vi "DF_conveyer_belt_control.vi"() -> ()   [LabVIEW 2019]
uses:
  LabVIEW_LJM/FoamWood/Control 3.ctl
  <vilib>/Instr/_visa.llb/VISA Configure Serial Port (Instr).vi
panel:
  in  "stop":bool
  in  "Speed (Hz)":T1=-5.5 step=0.1 format="%#_4g"
  in  "COM port":refnum<visa-resource-name>="COM7"
  out "error out":errorcluster={"status"=FALSE, "code"=1073676294, "source"="VISA Read in DF_conveyer_belt_control.vi"}
  # "Speed of the conveyer belt. The sign define the direction of the rotation."
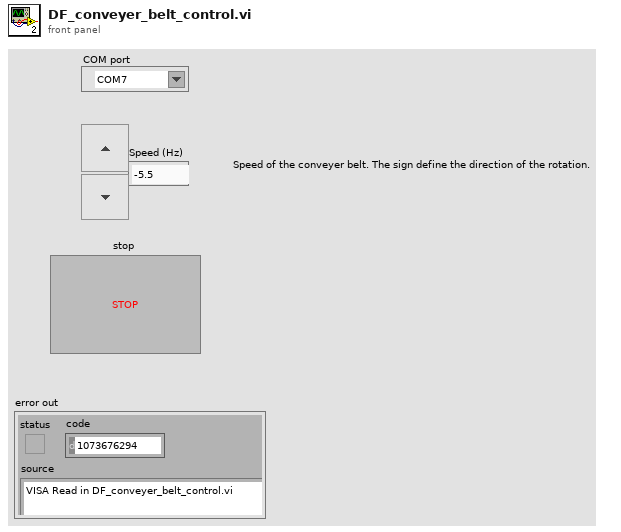
[diagram p1: front panel]
types:
  T1 = typedef "Control 3.ctl" = dbl
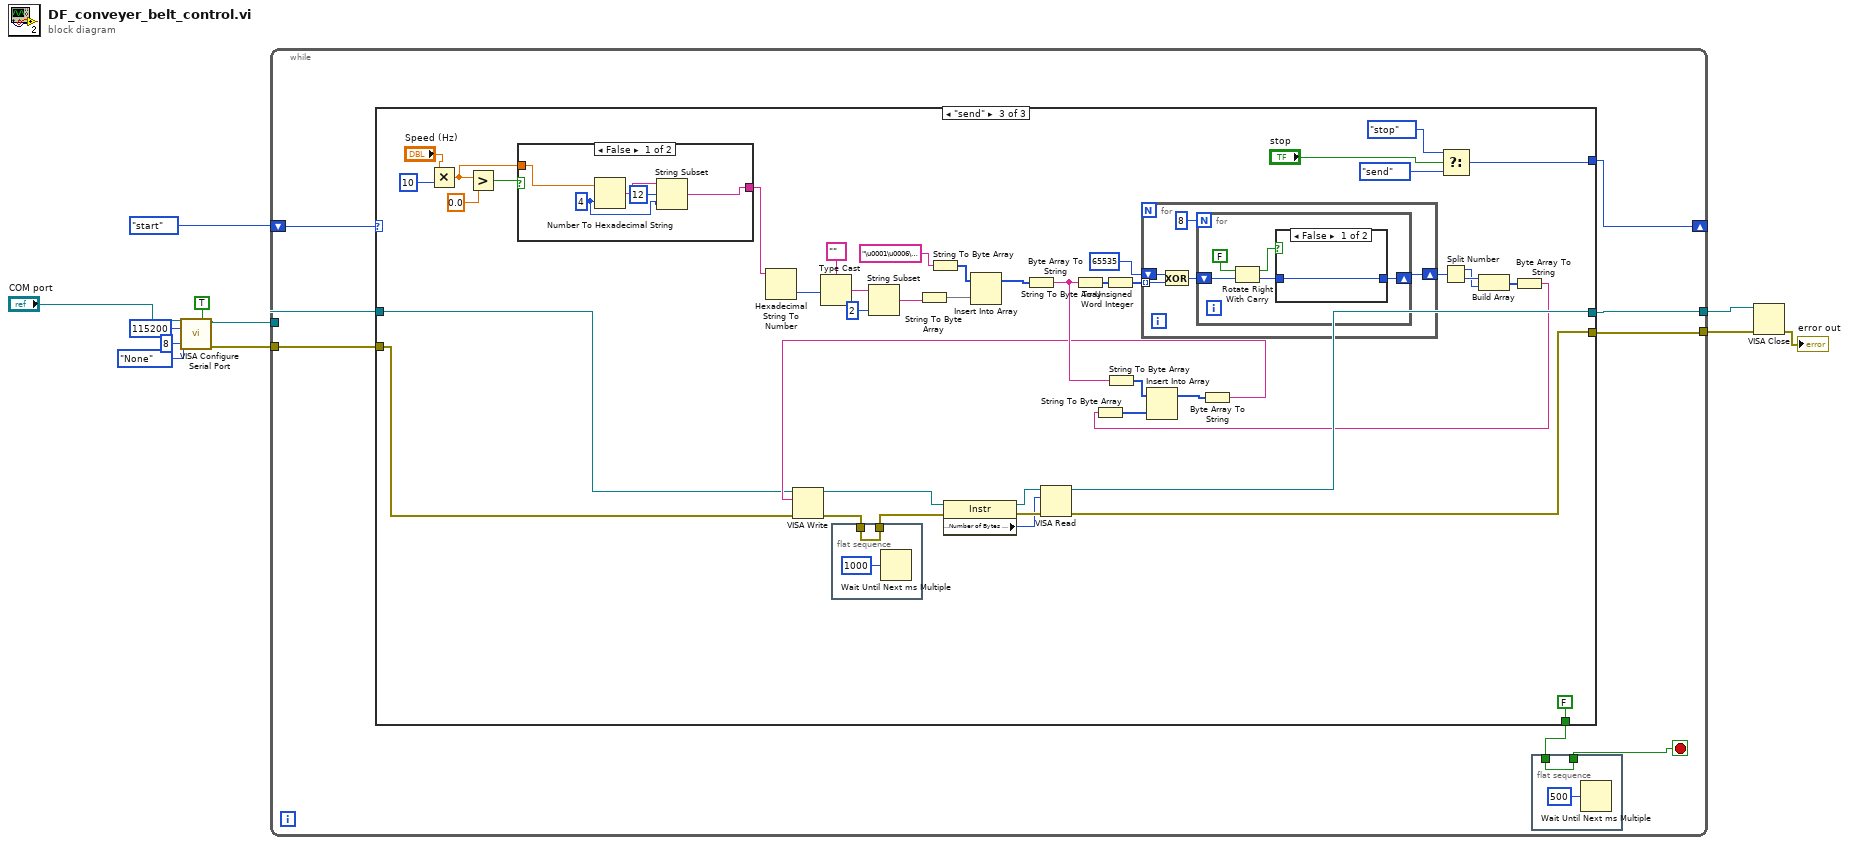
[diagram p0: block diagram]
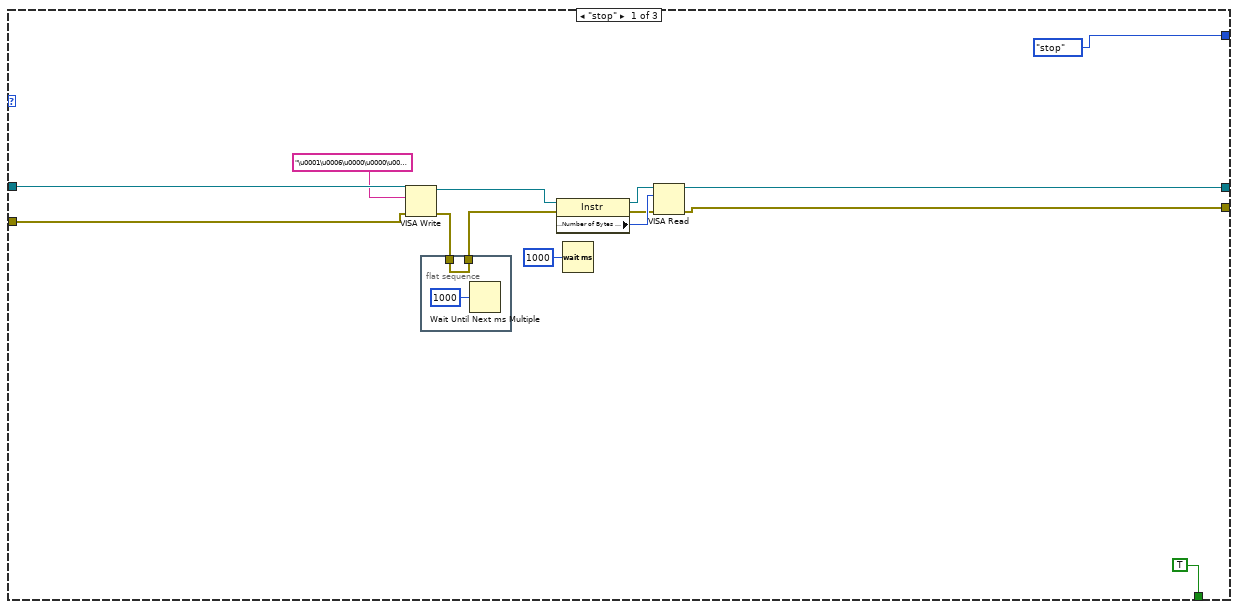
[diagram p2: hidden frame]
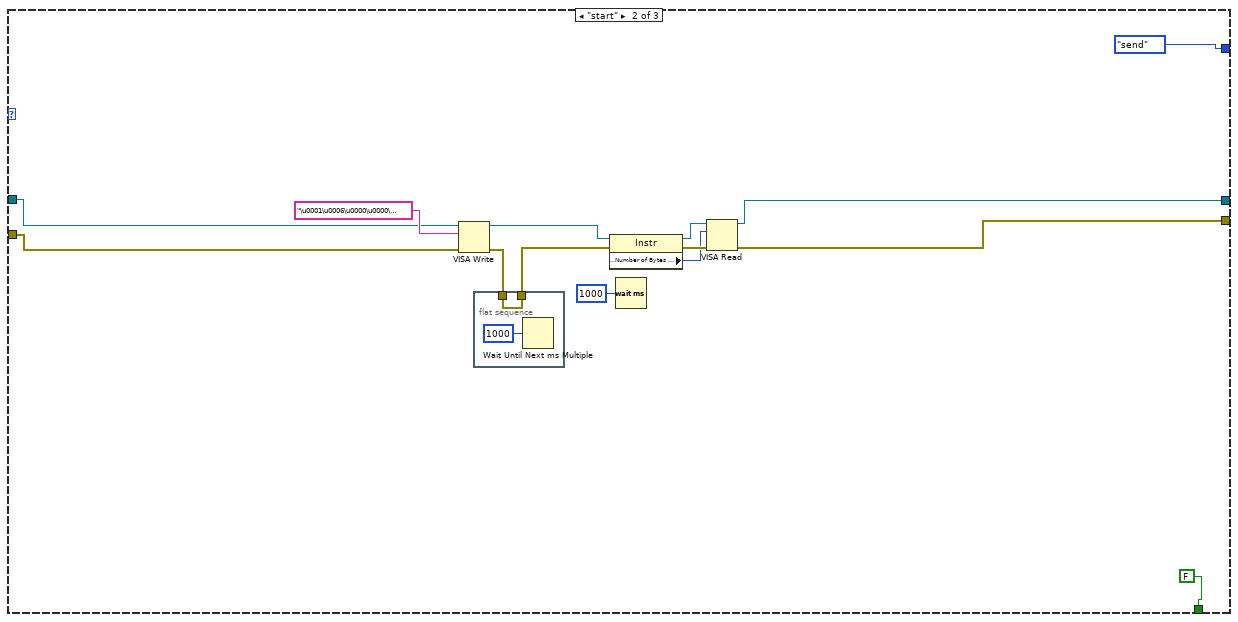
[diagram p3: hidden frame]
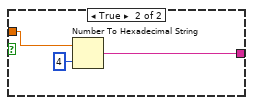
[diagram p4: hidden frame]
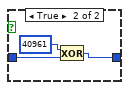
[diagram p5: hidden frame]
diagram:
  n1 = call-poly "VISA Configure Serial Port"("VISA resource name"="COM port", "Enable Termination\nChar (T)"=TRUE ("Enable Termination\nChar (T)"), "baud rate (9600)"=u32 115200, "data bits (8)"=u16 8, "parity (0:none)"=enum16{"None", "Odd", "Even", "Mark", "Space"}."None") -> ("VISA resource name out"=w6:refnum<visa-resource-name>, "error out"=w5:errorcluster)  [unwired: 2 in, 7 out]
  n2 = while {
    tunnel: [w16] -> w9
    tunnel: [w17] -> w8
    tunnel: w6 -> [w18]
    tunnel: w5 -> [w19]
    shift-right: [w15] -> _
    shift-left: enum16{"stop", "start", "send"}."start" -> [w14]
    stop <- w12 stop-if-true
    n3 = case shown="\"send\"" w14 {
      tunnel: w18 -> [w31 w43 w66]
      tunnel: w19 -> [w30 w42 w65]
      tunnel: [w28 w40 w89] -> w16
      tunnel: [w29 w41 w90] -> w17
      tunnel: [enum16{"stop", "start", "send"}."stop" enum16{"stop", "start", "send"}."send" w62] -> w15
      tunnel: [TRUE FALSE FALSE] -> w13
      frame "stop" {
        n4 = VISA Write(VISA resource name=w31, write buffer="\u0001\u0006\u0000\u0000\u0000\u0000‰Ê" ("write buffer (\"\")"), error in (no error)=w30) -> (VISA resource name out=w33:refnum<visa-resource-name>, error out=w25:errorcluster)  [unwired: 1 out]
        n5 = flat-sequence {
          tunnel: [w36] -> w24
          tunnel: w25 -> [w36]
          frame #0 {
            n6 = Wait Until Next ms Multiple(millisecond multiple=u32 1000) -> ()  [unwired: 1 out]
          }
        }
        n7 = property on="Property Node" class="Instr"(reference=w33, error in=w24) -> (reference out=w34:refnum<visa-resource-name>, error out=w32:errorcluster, "Serial Settings:Number of Bytes at Serial Port"=w35:u32)
        n8 = Wait (ms)(milliseconds to wait=u32 1000) -> ()  [unwired: 1 out]
        n9 = VISA Read(VISA resource name=w34, byte count=w35, error in (no error)=w32) -> (VISA resource name out=w29:refnum<visa-resource-name>, error out=w28:errorcluster)  [unwired: 2 out]
      }
      frame "start" {
        n10 = VISA Write(VISA resource name=w43, write buffer="\u0001\u0006\u0000\u0000\u0000\u0001H\n" ("write buffer (\"\")"), error in (no error)=w42) -> (VISA resource name out=w48:refnum<visa-resource-name>, error out=w50:errorcluster)  [unwired: 1 out]
        n11 = flat-sequence {
          tunnel: [w52] -> w51
          tunnel: w50 -> [w52]
          frame #0 {
            n12 = Wait Until Next ms Multiple(millisecond multiple=u32 1000) -> ()  [unwired: 1 out]
          }
        }
        n13 = property on="Property Node" class="Instr"(reference=w48, error in=w51) -> (reference out=w47:refnum<visa-resource-name>, error out=w49:errorcluster, "Serial Settings:Number of Bytes at Serial Port"=w46:u32)
        n14 = Wait (ms)(milliseconds to wait=u32 1000) -> ()  [unwired: 1 out]
        n15 = VISA Read(VISA resource name=w47, byte count=w46, error in (no error)=w49) -> (VISA resource name out=w41:refnum<visa-resource-name>, error out=w40:errorcluster)  [unwired: 2 out]
      }
      frame "send" {
        n16 = Multiply(x="Speed (Hz)", y=10) -> (x*y=w55:T1)
        n17 = Greater?(x=w55, y=T1 0.0) -> (0:w56:bool)
        n18 = case shown="False" w56 {
          tunnel: w55 -> [w100 w103]
          tunnel: [w99 w102] -> w54
          frame False {
            w98 = i16 4 ("width (-)")
            n19 = Number To Hexadecimal String(1:w98, 2:w100) -> (0:w101:string)
            n20 = String Subset(string=w101, offset (0)=12, length (rest)=w98) -> (substring=w99:string)
          }
          frame True {
            n21 = Number To Hexadecimal String(1:i16 4 ("width (-)"), 2:w103) -> (0:w102:string)
          }
        }
        n22 = Hexadecimal String To Number(string=w54) -> (number=w77:u32)  [unwired: 2 in, 1 out]
        n23 = Type Cast(type="" ("write buffer (\"\")"), x=w77) -> (*(type *) &x=w75:string)
        n24 = flat-sequence {
          tunnel: [w119] -> w92
          tunnel: w91 -> [w119]
          frame #0 {
            n25 = Wait Until Next ms Multiple(millisecond multiple=u32 1000) -> ()  [unwired: 1 out]
          }
        }
        n26 = String Subset(string=w75, offset (0)=2) -> (substring=w73:string)  [unwired: 1 in]
        n27 = String To Byte Array(string=w73) -> (unsigned byte array=w80:u8[])
        n28 = String To Byte Array(string="\u0001\u0006\u0000\u0001" ("write buffer (\"\")")) -> (unsigned byte array=w81:u8[])
        n29 = Insert Into Array(array=w81, new element=w80) -> (w79:u8[])  [unwired: 1 in]
        n30 = Byte Array To String(unsigned byte array=w79) -> (string=w69:string)
        n31 = String To Byte Array(string=w69) -> (unsigned byte array=w86:u8[])
        n32 = To Unsigned Word Integer(number=w86) -> (unsigned 16bit integer=w85:u16[])
        n33 = String To Byte Array(string=w69) -> (unsigned byte array=w72:u8[])
        n34 = for {
          shift-right: [w106] -> w87
          shift-left: u16 65535 -> [w107]
          tunnel: w85 -> [w105] mode=indexing
          n35 = Exclusive Or(1:w105, 2:w107) -> (0:w108:u16)
          n36 = for {
            N: 8 -> [_]
            shift-right: [w113] -> w106
            shift-left: w108 -> [w112]
            n37 = Rotate Right With Carry(2:w112, 3:FALSE ("Übertrag")) -> (0:w114:u16, 1:w111:bool)
            n38 = case shown="False" w111 {
              tunnel: w114 -> [w115 w117]
              tunnel: [w115 w116] -> w113
              frame False {
              }
              frame True {
                n39 = Exclusive Or(1:w117, 2:u16 40961) -> (0:w116:u16)
              }
            }
          }
        }
        n40 = Select(t=enum16{"stop", "start", "send"}."stop", s="stop", f=enum16{"stop", "start", "send"}."send") -> (s? t:f=w62:enum16{"stop", "start", "send"})
        n41 = Split Number(x=w87) -> (hi(x)=w83:u8, lo(x)=w84:u8)
        n42 = Build Array(w84, w83) -> (w82:u8[])
        n43 = Byte Array To String(unsigned byte array=w82) -> (string=w68:string)
        n44 = String To Byte Array(string=w68) -> (unsigned byte array=w71:u8[])
        n45 = Insert Into Array(array=w72, new element=w71) -> (w70:u8[])  [unwired: 1 in]
        n46 = Byte Array To String(unsigned byte array=w70) -> (string=w67:string)
        n47 = VISA Write(VISA resource name=w66, write buffer=w67, error in (no error)=w65) -> (VISA resource name out=w95:refnum<visa-resource-name>, error out=w91:errorcluster)  [unwired: 1 out]
        n48 = property on="Property Node" class="Instr"(reference=w95, error in=w92) -> (reference out=w94:refnum<visa-resource-name>, error out=w96:errorcluster, "Serial Settings:Number of Bytes at Serial Port"=w93:u32)
        n49 = VISA Read(VISA resource name=w94, byte count=w93, error in (no error)=w96) -> (VISA resource name out=w90:refnum<visa-resource-name>, error out=w89:errorcluster)  [unwired: 2 out]
      }
    }
    n50 = flat-sequence {
      tunnel: w13 -> [w20]
      tunnel: [w20] -> w12
      frame #0 {
        n51 = Wait Until Next ms Multiple(millisecond multiple=u32 500) -> ()  [unwired: 1 out]
      }
    }
  }
  n52 = VISA Close(VISA resource name=w8, error in (no error)=w9) -> (error out=→"error out":errorcluster)
